vi "Find Best Solution In Population.vi"(9 "Population Size":u8, 11 "Population":T2[](array[typedef])) -> (2 "Statistics Out":T1, 3 "Best Solution In Population":T2)   [LabVIEW 2013, in "GA.lvclass"]
uses:
  GA.lvclass
  GA_Class/Controls/Solution.ctl
  GA_Class/Controls/Population Statistics.ctl
  <vilib>/Analysis/baseanly.llb/Mean (DBL).vi
  <vilib>/Analysis/NI_AALBase.lvlib
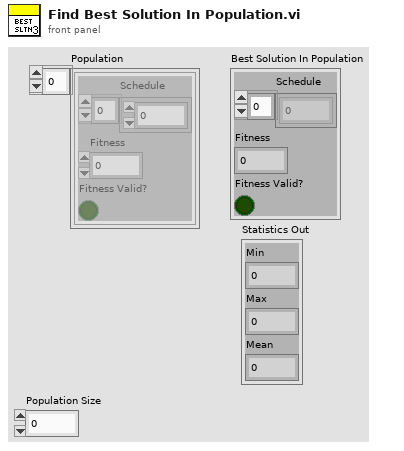
[diagram p1: front panel]
types:
  T1 = typedef "Population Statistics.ctl" = cluster{"Min":u16, "Max":u16, "Mean":dbl}
  T2 = typedef "Solution.ctl" = cluster{"Schedule":u16[], "Fitness":u16, "Fitness Valid?":bool}
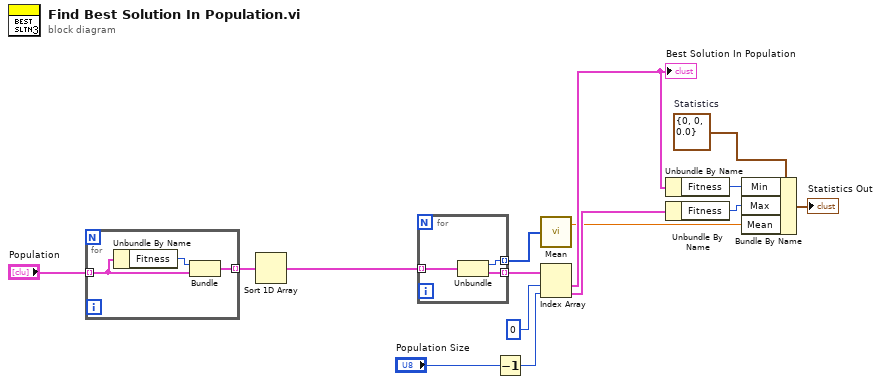
[diagram p0: block diagram]
diagram:
  w10 = T1 {"Min"=0, "Max"=0, "Mean"=0.0}  # Statistics
  n1 = for {
    tunnel: "Population" -> [w17] mode=indexing
    tunnel: [w16] -> w14 mode=indexing
    n2 = Unbundle By Name(w17) -> ("Fitness"=w18:u16)
    n3 = Bundle("Fitness"=w18, "Solution"=w17) -> (w16:cluster{"Fitness":u16, "Solution":T2})  [unwired: 1 in]
  }
  n4 = Sort 1D Array(array=w14) -> (sorted array=w13:cluster{"Fitness":u16, "Solution":T2}[])
  n5 = for {
    tunnel: w13 -> [w21] mode=indexing
    tunnel: [w20] -> w12 mode=indexing
    tunnel: [w19] -> w4 mode=indexing
    n6 = Unbundle(w21) -> ("Fitness"=w19:u16, "Solution"=w20:T2)
  }
  n7 = Decrement(x="Population Size") -> (x-1=w1:u8)
  n8 = call-poly <vilib>:"Mean.vi"("X"=w4) -> ("mean"=w3:dbl)  [unwired: 1 out]
  n9 = Index Array(array=w12, index #1=0 ("index"), index #2=w1) -> (element #1=w9:T2, element #2=w7:T2)
  "Best Solution In Population" <- w9
  n10 = Unbundle By Name(w9) -> ("Fitness"=w8:u16)
  n11 = Unbundle By Name(w7) -> ("Fitness"=w6:u16)
  n12 = Bundle By Name(cluster=w10, "Min"=w8, "Max"=w6, "Mean"=w3) -> (→"Statistics Out":T1)
